vi "produce_data.vi"(8 "error in (no error)":errorcluster, 9 "aData Out":dbl[][](array[numeric]), 10 "Queues":T1, 11 "Loop Data In":T2[](array[typedef])) -> (0 "error out":errorcluster, 3 "Loop Data Out":T2[](array[typedef]))   [LabVIEW 2025, in "LabJackEKG.lvlib"]
uses:
  LabJackEKG.lvlib
  Tests/StreamProducerLoopData.ctl
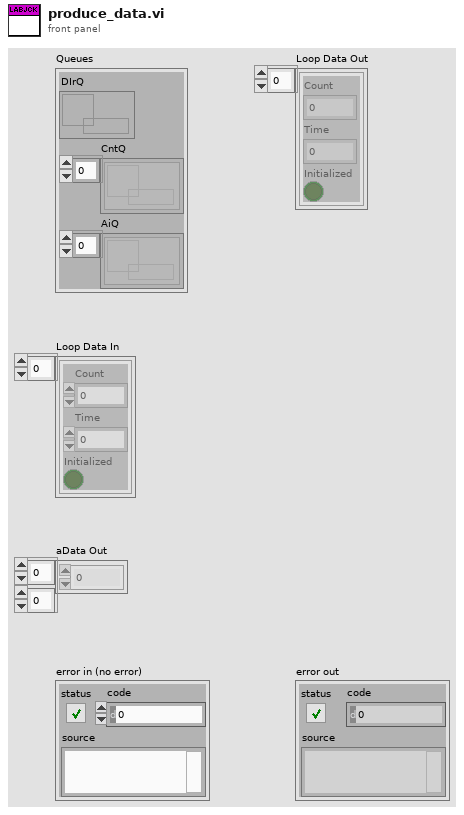
[diagram p1: front panel]
types:
  T1 = cluster{"DIrQ":refnum<queue>, "CntQ":refnum<queue>[], "AiQ":refnum<queue>[]}
  T2 = typedef "LabJackEKG.lvlib/StreamProducerLoopData.ctl" = cluster{"Count":i64, "Time":i64, "Initialized":bool}
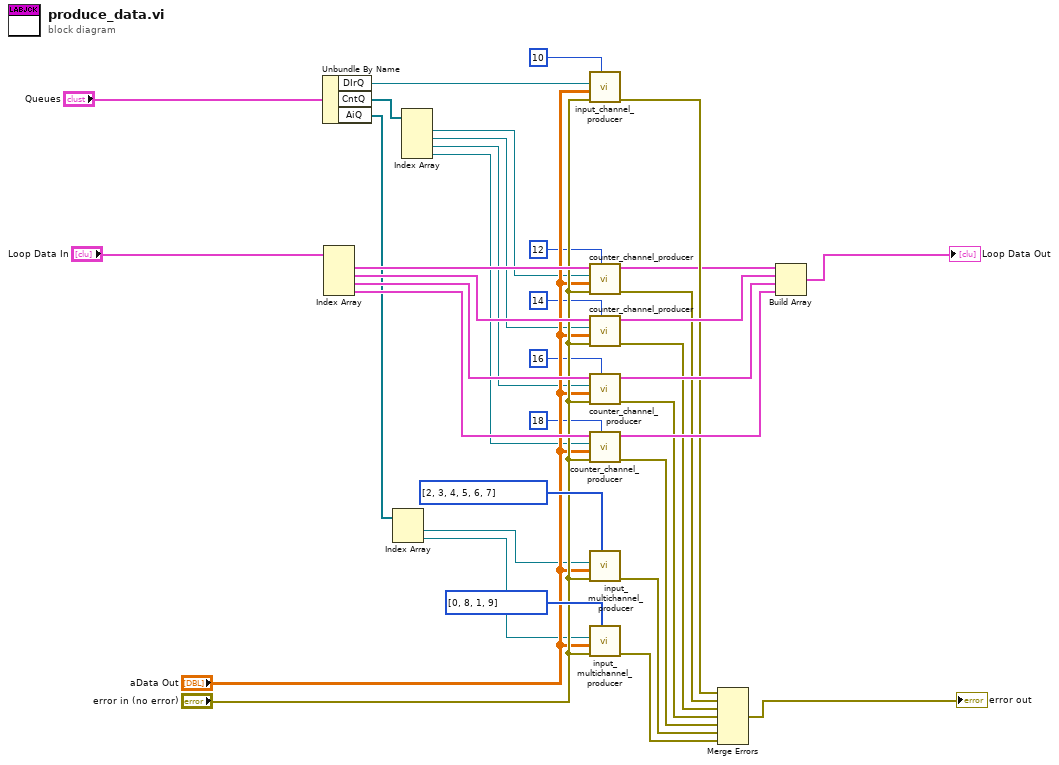
[diagram p0: block diagram]
diagram:
  n1 = Unbundle By Name("Queues") -> ("DIrQ"=w26:refnum<queue>, "CntQ"=w27:refnum<queue>[], "AiQ"=w28:refnum<queue>[])
  n2 = Index Array(array="Loop Data In") -> (element #1=w34:T2, element #2=w35:T2, element #3=w36:T2, element #4=w37:T2)  [unwired: 4 in]
  n3 = Index Array(array=w28) -> (element #1=w16:refnum<queue>, element #2=w17:refnum<queue>)  [unwired: 2 in]
  n4 = Index Array(array=w27) -> (element #1=w10:refnum<queue>, element #2=w11:refnum<queue>, element #3=w12:refnum<queue>, element #4=w13:refnum<queue>)  [unwired: 4 in]
  n5 = call "input_channel_producer.vi"("Index"=10 ("Channel"), "error in (no error)"="error in (no error)", "aData Out"="aData Out", "Q"=w26) -> ("error out"=w22:errorcluster)  [unwired: 7 in]
  n6 = call "counter_channel_producer.vi"("Channel"=12 ("disabled index (col)"), "error in (no error)"="error in (no error)", "aData Out"="aData Out", "Queue in"=w10, "output cluster in"=w34) -> ("error out"=w1:errorcluster, "output cluster out"=w2:T2)  [unwired: 5 in]
  n7 = call "counter_channel_producer.vi"("Channel"=14 ("disabled index"), "error in (no error)"="error in (no error)", "aData Out"="aData Out", "Queue in"=w11, "output cluster in"=w35) -> ("error out"=w5:errorcluster, "output cluster out"=w29:T2)  [unwired: 5 in]
  n8 = call "counter_channel_producer.vi"("Channel"=16 ("disabled index"), "error in (no error)"="error in (no error)", "aData Out"="aData Out", "Queue in"=w12, "output cluster in"=w36) -> ("error out"=w9:errorcluster, "output cluster out"=w30:T2)  [unwired: 5 in]
  n9 = call "counter_channel_producer.vi"("Channel"=18 ("disabled index"), "error in (no error)"="error in (no error)", "aData Out"="aData Out", "Queue in"=w13, "output cluster in"=w37) -> ("error out"=w8:errorcluster, "output cluster out"=w31:T2)  [unwired: 5 in]
  n10 = call "input_multichannel_producer.vi"("Indices"=i32[] [2, 3, 4, 5, 6, 7], "error in (no error)"="error in (no error)", "aData Out"="aData Out", "Q"=w16) -> ("error out"=w15:errorcluster)  [unwired: 7 in]
  n11 = call "input_multichannel_producer.vi"("Indices"=i32[] [0, 8, 1, 9], "error in (no error)"="error in (no error)", "aData Out"="aData Out", "Q"=w17) -> ("error out"=w18:errorcluster)  [unwired: 7 in]
  n12 = Merge Errors(w22, w1, w5, w9, w8, w15, w18) -> (→"error out":errorcluster)
  n13 = Build Array(w2, w29, w30, w31) -> (→"Loop Data Out":T2[])
